vi "Get AO Data Value.vi"(8 "error in (no error)":errorcluster, 10 "AO IOName":string, 11 "DAQ":refnum<class "DAQ.lvclass">) -> (0 "error out":errorcluster, 2 "Value":dbl, 3 "DAQ":refnum<class "DAQ.lvclass">)   [LabVIEW 2017, in "DAQ.lvclass"]
doc: "Developed by Kevin Thompson\nkevin@thompsonengineering.net\n\nCopyright 2018-2020\nThompson Engineering, LLC"
uses:
  DAQ.lvclass
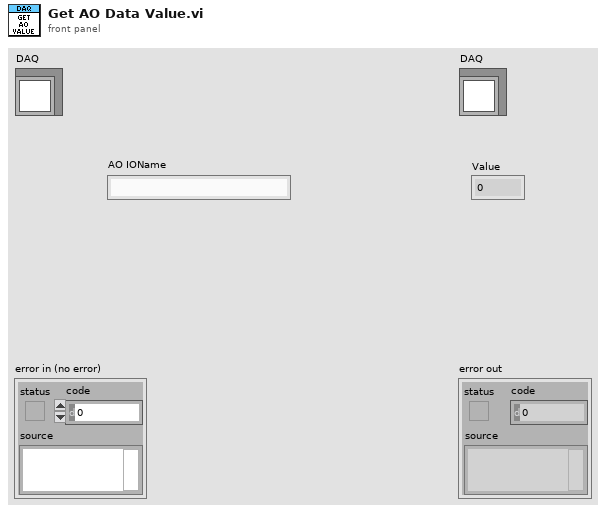
[diagram p1: front panel]
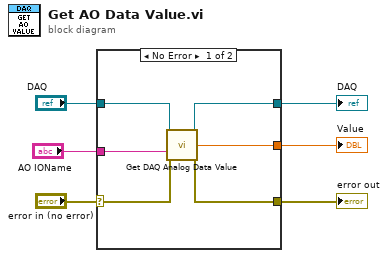
[diagram p0: block diagram]
diagram:
  n1 = case shown="No Error" "error in (no error)" {
    selector: "error in (no error)" -> [w11 w14]
    tunnel: [w10 w14] -> w5
    tunnel: [w8 w13] -> w3
    tunnel: "DAQ" -> [w9 w13]
    tunnel: [w12 _] -> w2
    tunnel: "AO IOName" -> [w7 _]
    frame No Error {
      n2 = call "Get DAQ Analog Data Value.vi"("DAQ"=w9, "Name"=w7, "error in (no error)"=w11) -> ("DAQ"=w8:refnum<class "DAQ.lvclass">, "Value"=w12:dbl, "error out"=w10:errorcluster)  [unwired: 10 in]
    }
    frame Error {
    }
  }
  "error out" <- w5
  "DAQ" <- w3
  "Value" <- w2
